vi "Setup multiple ramp in bipolar.vi"(4 "Channel Name (1)":u16(ring)=1 items=["1"=1, "2"=2, "3"=3, "4"=4], 5 "VISA resource name":refnum<visa-resource-name>="GPIB0::1::INSTR", 7 "End time S":dbl=0.000105, 8 "error in (no error)":errorcluster, 9 "Ramp time S":dbl=0.01, 10 "Delay time S":dbl=0.01, 11 "Sampling Frequency (Hz)":u64=10000000) -> (0 "error out":errorcluster)   [LabVIEW 2021]
uses:
  <vilib>/Waveform/DWDTOps.llb/DWDT Boolean Array to Digital.vi
  <instrlib>/Tektronix AWG 5000 7000 Series/Public/Configure/Channel/Assign Output Waveform (From Waveform List).vi
  <instrlib>/Tektronix AWG 5000 7000 Series/Public/Configure/Configure Output Timing (Sampling Frequency).vi
  <instrlib>/Tektronix AWG 5000 7000 Series/Tektronix AWG 5000 7000 Series.lvlib
panel:
  in  "Ramp time S 3":dbl=0.01
  in  "Ramp time S 2":dbl=0.02
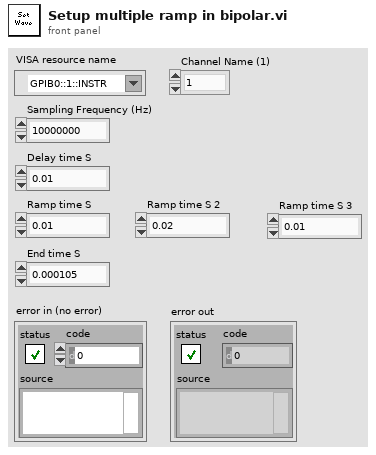
[diagram p1: front panel]
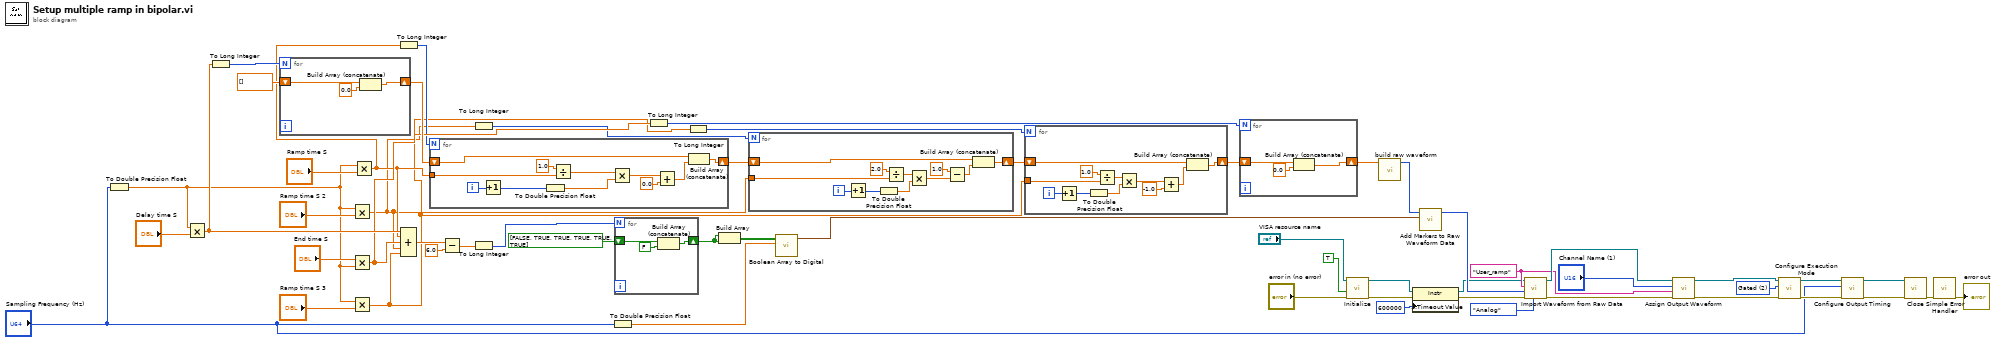
[diagram p0: block diagram]
diagram:
  w28 = u16 2 items=["Continuous", "Triggered", "Gated", "Sequence", "Triggered Continuous"] ("Execution Mode (0 : Continuous)")
  w30 = "User_ramp" ("Waveform Name")
  n1 = To Double Precision Float(number="Sampling Frequency (Hz)") -> (double precision float=w5:dbl)
  n2 = Multiply(x=w5, y="Delay time S") -> (x*y=w38:dbl)
  n3 = To Long Integer(number=w38) -> (32bit integer=w25:i32)
  n4 = for {
    N: w25 -> [_]
    shift-right: [w58] -> w44
    shift-left: dbl[] [] -> [w59]
    n5 = Build Array (concatenate)(w59, 0.0) -> (w58:dbl[])
  }
  n6 = Multiply(x=w5, y="Ramp time S 2") -> (x*y=w9:dbl)
  n7 = Multiply(x="End time S", y=w5) -> (x*y=w37:dbl)
  n8 = Multiply(x=w5, y="Ramp time S 3") -> (x*y=w1:dbl)
  n9 = Multiply(x=w5, y="Ramp time S") -> (x*y=w10:dbl)
  n10 = To Long Integer(number=w10) -> (32bit integer=w24:i32)
  n11 = Compound Arithmetic op=ADD(w38, w10, w37, w9, w1) -> (w36:dbl)
  n12 = for {
    N: w24 -> [_]
    shift-right: [w62] -> w11
    shift-left: w44 -> [w64]
    tunnel: w10 -> [w61]
    i -> [w68]
    n13 = Increment(x=w68) -> (x+1=w67:i32)
    n14 = To Double Precision Float(number=w67) -> (double precision float=w60:dbl)
    n15 = Divide(x=1.0, y=w61) -> (x/y=w69:dbl)
    n16 = Multiply(x=w69, y=w60) -> (x*y=w66:dbl)
    n17 = Add(x=w66, y=0.0) -> (x+y=w63:dbl)
    n18 = Build Array (concatenate)(w64, w63) -> (w62:dbl[])
  }
  n19 = Subtract(x=w36, y=6.0) -> (x-y=w34:dbl)
  n20 = To Long Integer(number=w9) -> (32bit integer=w8:i32)
  n21 = To Long Integer(number=w34) -> (32bit integer=w26:i32)
  n22 = To Double Precision Float(number="Sampling Frequency (Hz)") -> (double precision float=w13:dbl)
  n23 = for {
    N: w26 -> [_]
    shift-right: [w71] -> w15
    shift-left: bool[] [FALSE, TRUE, TRUE, TRUE, TRUE, TRUE] -> [w73]
    n24 = Build Array (concatenate)(w73, FALSE) -> (w71:bool[])
  }
  n25 = To Long Integer(number=w37) -> (32bit integer=w7:i32)
  n26 = To Long Integer(number=w1) -> (32bit integer=w4:i32)
  n27 = Build Array(w15, w15) -> (w33:bool[][])
  n28 = for {
    N: w8 -> [_]
    shift-right: [w83] -> w3
    shift-left: w11 -> [w84]
    tunnel: w9 -> [w82]
    i -> [w80]
    n29 = Increment(x=w80) -> (x+1=w79:i32)
    n30 = To Double Precision Float(number=w79) -> (double precision float=w77:dbl)
    n31 = Divide(x=2.0, y=w82) -> (x/y=w78:dbl)
    n32 = Multiply(x=w78, y=w77) -> (x*y=w75:dbl)
    n33 = Subtract(x=1.0, y=w75) -> (x-y=w74:dbl)
    n34 = Build Array (concatenate)(w84, w74) -> (w83:dbl[])
  }
  n35 = call-poly <vilib>:"Boolean Array to Digital.vi"("sample rate"=w13, "boolean array"=w33) -> ("digital waveform"=w22:digitalwaveform)  [unwired: 8 in, 1 out]
  n36 = for {
    N: w4 -> [_]
    shift-right: [w85] -> w2
    shift-left: w3 -> [w95]
    tunnel: w1 -> [w92]
    i -> [w94]
    n37 = Increment(x=w94) -> (x+1=w90:i32)
    n38 = To Double Precision Float(number=w90) -> (double precision float=w89:dbl)
    n39 = Divide(x=1.0, y=w92) -> (x/y=w91:dbl)
    n40 = Multiply(x=w91, y=w89) -> (x*y=w88:dbl)
    n41 = Add(x=w88, y=-1.0) -> (x+y=w86:dbl)
    n42 = Build Array (concatenate)(w95, w86) -> (w85:dbl[])
  }
  n43 = for {
    N: w7 -> [_]
    shift-right: [w97] -> w40
    shift-left: w2 -> [w98]
    n44 = Build Array (concatenate)(w98, 0.0) -> (w97:dbl[])
  }
  n45 = call <instrlib>:"Initialize.vi"("error in (no error)"="error in (no error)", "Reset (False)"=TRUE ("Reset? (F: No)"), "VISA resource name"="VISA resource name") -> ("error out"=w17:errorcluster, "VISA resource name out"=w19:refnum<visa-resource-name>)  [unwired: 7 in]
  n46 = call "build raw waveform.vi"("Y"=w40) -> ("Raw Waveform Data"=w23:u8[])  [unwired: 10 in]
  n47 = property class="Instr"(reference=w19, error in=w17, "General Settings:Timeout Value"=u32 600000) -> (reference out=w18:refnum<visa-resource-name>, error out=w16:errorcluster)
  n48 = call <instrlib>:"Add Markers to Raw Waveform Data.vi"("Markers"=w22, "Raw Waveform Data"=w23) -> ("Raw Waveform Data with Markers"=w21:u8[])  [unwired: 9 in]
  n49 = call <instrlib>:"Import Waveform from Raw Data.vi"("Representation (1 : Analog)"=enum16{"Integer", "Analog"}."Analog", "error in (no error)"=w16, "Raw Data"=w21, "Waveform Name"=w30, "VISA resource name"=w18) -> ("error out"=w29:errorcluster, "VISA resource name out"=w31:refnum<visa-resource-name>)  [unwired: 5 in]
  n50 = call-poly <instrlib>:"Assign Output Waveform.vi"("error in (no error)"=w29, "Waveform"=w30, "Channel Name (1)"="Channel Name (1)", "VISA resource name"=w31) -> ("error out"=w54:errorcluster, "VISA resource name out"=w55:refnum<visa-resource-name>)  [unwired: 6 in]
  n51 = call <instrlib>:"Configure Execution Mode.vi"("error in (no error)"=w54, "Execution Mode (0 : Continuous)"=w28, "VISA resource name"=w55) -> ("error out"=w52:errorcluster, "VISA resource name out"=w53:refnum<visa-resource-name>)  [unwired: 7 in]
  n52 = call-poly <instrlib>:"Configure Output Timing.vi"("error in (no error)"=w52, "Sampling Frequency (Hz) (100MHz)"="Sampling Frequency (Hz)", "VISA resource name"=w53) -> ("error out"=w50:errorcluster, "VISA resource name out"=w51:refnum<visa-resource-name>)  [unwired: 7 in]
  n53 = call <instrlib>:"Close.vi"("error in (no error)"=w50, "VISA resource name"=w51) -> ("error out"=w49:errorcluster)  [unwired: 9 in]
  n54 = call <vilib>:"Simple Error Handler.vi"("error in (no error)"=w49) -> ("error out"=→"error out":errorcluster)  [unwired: 4 in, 4 out]
